vi "getConfig_summaryState.vi"(8 "error in (no error)":errorcluster) -> (0 "error out":errorcluster, 2 "priority":i32, 3 "summaryState":i32)   [LabVIEW 2018]
doc: "Get the configuration of summary state."
uses:
  <vilib>/Utility/config.llb/Read Key (I32).vi
  <vilib>/Utility/config.llb/NI_LVConfig.lvlib
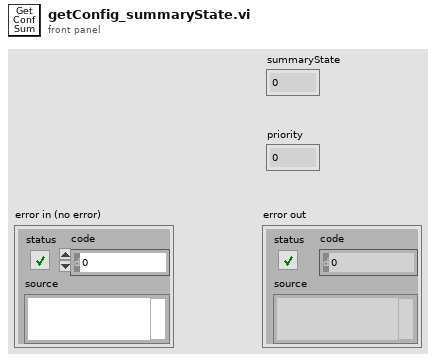
[diagram p1: front panel]
types:
  T1 = typedef "NI_LVConfig.lvlib/Config Data RefNum.ctl" = refnum<k1>
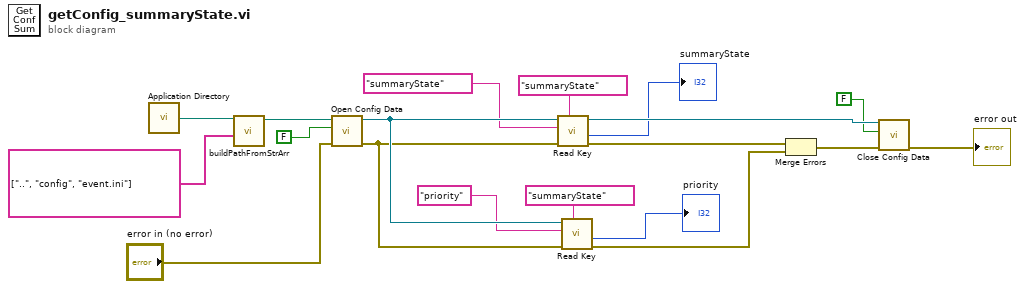
[diagram p0: block diagram]
diagram:
  n1 = call <vilib>:"Application Directory.vi"() -> ("Application Directory"=w19:path)
  n2 = call "buildPathFromStrArr.vi"("String Array"=string[] ["..", "config", "event.ini"], "Root Path"=w19) -> ("Absolute Path"=w17:path)  [unwired: 9 in]
  n3 = call <vilib>:"Open Config Data.vi"("error in (no error)"="error in (no error)", "create file if necessary (T)"=FALSE, "configuration file path"=w17) -> ("error out"=w13:errorcluster, "refnum"=w14:T1)  [unwired: 6 in, 1 out]
  n4 = call-poly <vilib>:"Read Key.vi"("section"="summaryState", "error in (no error)"=w13, "key"="summaryState", "refnum"=w14) -> ("error out"=w10:errorcluster, "value"=→"summaryState":i32, "refnum out"=w7:T1)  [unwired: 4 in, 1 out]
  n5 = call-poly <vilib>:"Read Key.vi"("section"="summaryState", "error in (no error)"=w13, "key"="priority", "refnum"=w14) -> ("error out"=w9:errorcluster, "value"=→"priority":i32)  [unwired: 4 in, 2 out]
  n6 = Merge Errors(w10, w9) -> (w8:errorcluster)
  n7 = call <vilib>:"Close Config Data.vi"("error in (no error)"=w8, "write file if changed (T)"=FALSE, "refnum"=w7) -> ("error out"=→"error out":errorcluster)  [unwired: 7 in, 1 out]
